vi "MC INIT Mixed Mode.vi"(8 "error in (no error)":errorcluster, 11 "MC VISA resource in":refnum<visa-resource-name>="ASRL1::INSTR") -> (0 "MC error out":errorcluster, 1 "MC Init Complete":bool, 3 "MC VISA resource  out":refnum<visa-resource-name>)   [LabVIEW 2009]
uses:
  <vilib>/Instr/_visa.llb/VISA Configure Serial Port (Instr).vi
panel:
  out "All Stop":bool
  out "Set Mode 3":bool
  in  "Mode command 3":string="^04 C0"
  out "Set Mode 2":bool
  in  "Mode command 2":string="^03 00"
  out "Set RS232 Control":bool
  out "Set Mode 1":bool
  in  "Mode command 1":string="^01 C5"
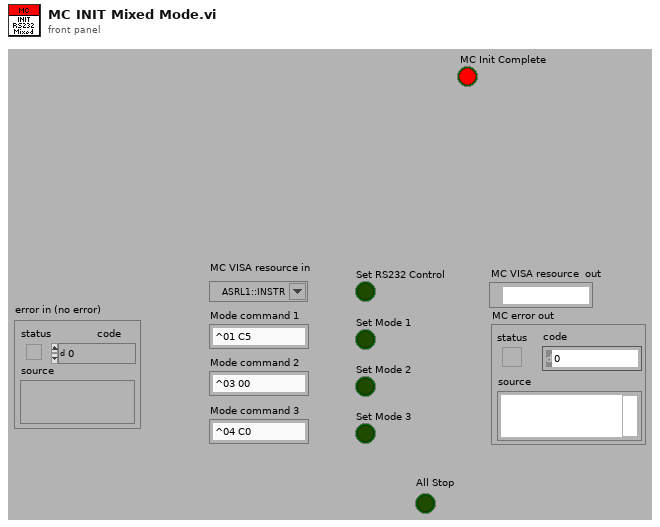
[diagram p1: front panel]
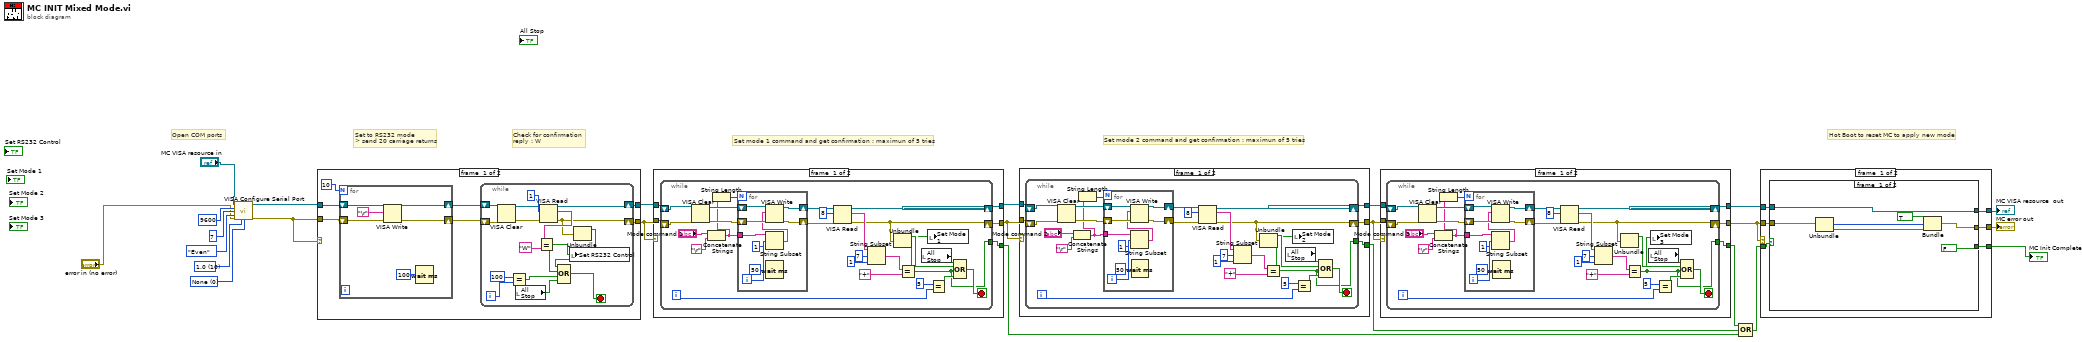
[diagram p0: block diagram]
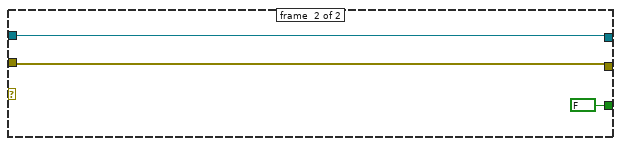
[diagram p2: hidden frame]
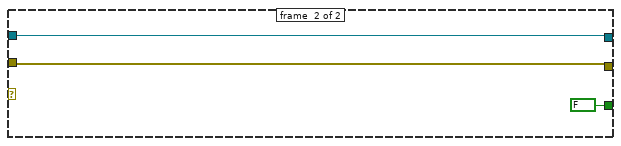
[diagram p3: hidden frame]
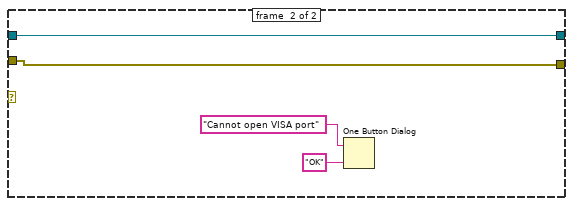
[diagram p4: hidden frame]
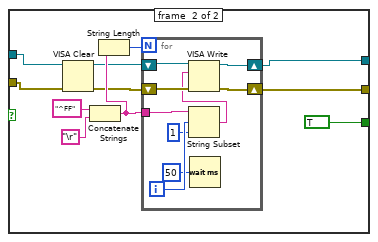
[diagram p5: hidden frame]
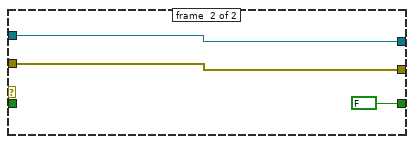
[diagram p6: hidden frame]
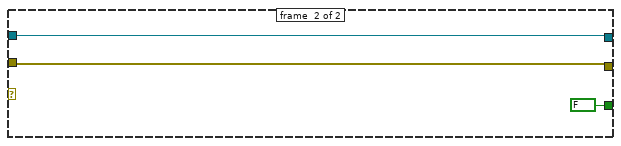
[diagram p7: hidden frame]
diagram:
  w20 = u16 0 items=["None", "XON/XOFF", "RTS/CTS", "XON/XOFF & RTS/CTS", "DTR/DSR", "XON/XOFF & DTR/DSR"] ("flow control (0:none)")
  w21 = u16 10 items=["1.0"=10, "1.5"=15, "2.0"=20] ("stop bits (10: 1 bit)")
  # "Set mode 2 command and get confirmation : maximun of 5 tries"
  # "Hot Boot to reset MC to apply new mode"
  # "Check for confirmation\nreply : W"
  # "Set mode 1 command and get confirmation : maximun of 5 tries"
  # "Set to RS232 mode\n> send 20 carriage returns"
  # "Open COM ports"
  n1 = call-poly "VISA Configure Serial Port"("VISA resource name"="MC VISA resource in", "baud rate (9600)"=u32 9600, "data bits (8)"=u16 7, "parity (0:none)"=enum16{"None", "Odd", "Even", "Mark", "Space"}."Even", "error in (no error)"="error in (no error)", "stop bits (10: 1 bit)"=w21, "flow control (0:none)"=w20) -> ("VISA resource name out"=w19:refnum<visa-resource-name>, "error out"=w15:errorcluster)  [unwired: 7 out]
  n2 = case shown="No Error" w15 {
    tunnel: w15 -> [w30 w56]
    tunnel: w19 -> [w29 w57]
    tunnel: [w28 w57] -> w18
    tunnel: [w25 w56] -> w16
    frame #0 {
      n3 = for {
        N: 10 -> [_]
        shift-right: [w50] -> w27
        shift-left: w30 -> [w53]
        shift-right: [w52] -> w26
        shift-left: w29 -> [w51]
        n4 = VISA Write(VISA resource name=w51, write buffer="\r", error in (no error)=w53) -> (VISA resource name out=w52:refnum<visa-resource-name>, error out=w50:errorcluster)  [unwired: 1 out]
        n5 = Wait (ms)(milliseconds to wait=u32 100) -> ()  [unwired: 1 out]
      }
      n6 = while {
        shift-right: [w43] -> w28
        shift-left: w26 -> [w44]
        shift-right: [w35] -> w25
        shift-left: w27 -> [w42]
        i -> [w39]
        stop <- w36 stop-if-true
        n7 = VISA Clear(VISA resource name=w44, error in (no error)=w42) -> (VISA resource name out=w41:refnum<visa-resource-name>, error out=w34:errorcluster)
        n8 = Equal?(x=100, y=w39) -> (x = y?=w37:bool)
        n9 = local read "All Stop"() -> (w32:bool)
        n10 = VISA Read(VISA resource name=w41, byte count=u32 1, error in (no error)=w34) -> (VISA resource name out=w43:refnum<visa-resource-name>, read buffer=w46:string, error out=w35:errorcluster)  [unwired: 1 out]
        n11 = Equal?(x=w46, y="W") -> (x = y?=w33:bool)
        n12 = local write "Set RS232 Control"(w33) -> ()
        n13 = Unbundle(w35) -> ("status"=w40:bool)  [unwired: 2 out]
        n14 = Compound Arithmetic op=OR(w40, w33, w37, w32) -> (w36:bool)
      }
    }
    frame #1 {
      n15 = One Button Dialog(message="Cannot open VISA port", button name ("OK")="OK") -> ()  [unwired: 1 out]
    }
  }
  n16 = case shown="No Error" w16 {
    tunnel: [w62 w99] -> w11
    tunnel: [w61 w98] -> w12
    tunnel: w18 -> [w60 w99]
    tunnel: w16 -> [w59 w98]
    tunnel: [w58 FALSE] -> w13
    frame #0 {
      n17 = while {
        shift-right: [w83] -> w62
        shift-left: w60 -> [w87]
        shift-right: [w70] -> w61
        shift-left: w59 -> [w86]
        tunnel: [w64] -> w58
        i -> [w67]
        stop <- w65 stop-if-true
        n18 = VISA Clear(VISA resource name=w87, error in (no error)=w86) -> (VISA resource name out=w80:refnum<visa-resource-name>, error out=w79:errorcluster)
        n19 = Concatenate Strings("Mode command 1", "\r") -> (w71:string)
        n20 = String Length(string=w71) -> (length=w72:i32)
        n21 = for {
          N: w72 -> [_]
          tunnel: w71 -> [w92]
          shift-right: [w96] -> w85
          shift-left: w79 -> [w93]
          shift-right: [w95] -> w84
          shift-left: w80 -> [w94]
          i -> [w91]
          n22 = String Subset(string=w92, offset (0)=w91, length (rest)=1 ("length (rest)")) -> (substring=w89:string)
          n23 = VISA Write(VISA resource name=w94, write buffer=w89, error in (no error)=w93) -> (VISA resource name out=w95:refnum<visa-resource-name>, error out=w96:errorcluster)  [unwired: 1 out]
          n24 = Wait (ms)(milliseconds to wait=u32 50) -> ()  [unwired: 1 out]
        }
        n25 = VISA Read(VISA resource name=w84, byte count=u32 8, error in (no error)=w85) -> (VISA resource name out=w83:refnum<visa-resource-name>, read buffer=w76:string, error out=w70:errorcluster)  [unwired: 1 out]
        n26 = String Subset(string=w76, offset (0)=7, length (rest)=1 ("length (rest)")) -> (substring=w75:string)
        n27 = Unbundle(w70) -> ("status"=w66:bool)  [unwired: 2 out]
        n28 = Equal?(x=w75, y="+") -> (x = y?=w64:bool)
        n29 = local read "All Stop"() -> (w63:bool)
        n30 = local write "Set Mode 1"(w64) -> ()
        n31 = Equal?(x=5, y=w67) -> (x = y?=w68:bool)
        n32 = Compound Arithmetic op=OR(w63, w66, w64, w68) -> (w65:bool)
      }
    }
    frame #1 {
    }
  }
  n33 = case shown="No Error" w12 {
    tunnel: [w104 w141] -> w9
    tunnel: [w103 w140] -> w8
    tunnel: w11 -> [w102 w141]
    tunnel: w12 -> [w101 w140]
    tunnel: [w100 FALSE] -> w10
    frame #0 {
      n34 = while {
        shift-right: [w125] -> w104
        shift-left: w102 -> [w129]
        shift-right: [w112] -> w103
        shift-left: w101 -> [w128]
        tunnel: [w106] -> w100
        i -> [w109]
        stop <- w107 stop-if-true
        n35 = VISA Clear(VISA resource name=w129, error in (no error)=w128) -> (VISA resource name out=w122:refnum<visa-resource-name>, error out=w121:errorcluster)
        n36 = Concatenate Strings("Mode command 2", "\r") -> (w113:string)
        n37 = String Length(string=w113) -> (length=w114:i32)
        n38 = for {
          N: w114 -> [_]
          tunnel: w113 -> [w134]
          shift-right: [w138] -> w127
          shift-left: w121 -> [w135]
          shift-right: [w137] -> w126
          shift-left: w122 -> [w136]
          i -> [w133]
          n39 = String Subset(string=w134, offset (0)=w133, length (rest)=1 ("length (rest)")) -> (substring=w131:string)
          n40 = VISA Write(VISA resource name=w136, write buffer=w131, error in (no error)=w135) -> (VISA resource name out=w137:refnum<visa-resource-name>, error out=w138:errorcluster)  [unwired: 1 out]
          n41 = Wait (ms)(milliseconds to wait=u32 50) -> ()  [unwired: 1 out]
        }
        n42 = VISA Read(VISA resource name=w126, byte count=u32 8, error in (no error)=w127) -> (VISA resource name out=w125:refnum<visa-resource-name>, read buffer=w118:string, error out=w112:errorcluster)  [unwired: 1 out]
        n43 = String Subset(string=w118, offset (0)=7, length (rest)=1 ("length (rest)")) -> (substring=w117:string)
        n44 = Unbundle(w112) -> ("status"=w108:bool)  [unwired: 2 out]
        n45 = Equal?(x=w117, y="+") -> (x = y?=w106:bool)
        n46 = local read "All Stop"() -> (w105:bool)
        n47 = local write "Set Mode 2"(w106) -> ()
        n48 = Equal?(x=5, y=w109) -> (x = y?=w110:bool)
        n49 = Compound Arithmetic op=OR(w105, w108, w106, w110) -> (w107:bool)
      }
    }
    frame #1 {
    }
  }
  n50 = case shown="No Error" w8 {
    tunnel: [w146 w183] -> w7
    tunnel: [w145 w182] -> w5
    tunnel: w9 -> [w144 w183]
    tunnel: w8 -> [w143 w182]
    tunnel: [w142 FALSE] -> w6
    frame #0 {
      n51 = while {
        shift-right: [w167] -> w146
        shift-left: w144 -> [w171]
        shift-right: [w154] -> w145
        shift-left: w143 -> [w170]
        tunnel: [w148] -> w142
        i -> [w151]
        stop <- w149 stop-if-true
        n52 = VISA Clear(VISA resource name=w171, error in (no error)=w170) -> (VISA resource name out=w164:refnum<visa-resource-name>, error out=w163:errorcluster)
        n53 = Concatenate Strings("Mode command 3", "\r") -> (w155:string)
        n54 = String Length(string=w155) -> (length=w156:i32)
        n55 = for {
          N: w156 -> [_]
          tunnel: w155 -> [w176]
          shift-right: [w180] -> w169
          shift-left: w163 -> [w177]
          shift-right: [w179] -> w168
          shift-left: w164 -> [w178]
          i -> [w175]
          n56 = String Subset(string=w176, offset (0)=w175, length (rest)=1 ("length (rest)")) -> (substring=w173:string)
          n57 = VISA Write(VISA resource name=w178, write buffer=w173, error in (no error)=w177) -> (VISA resource name out=w179:refnum<visa-resource-name>, error out=w180:errorcluster)  [unwired: 1 out]
          n58 = Wait (ms)(milliseconds to wait=u32 50) -> ()  [unwired: 1 out]
        }
        n59 = VISA Read(VISA resource name=w168, byte count=u32 8, error in (no error)=w169) -> (VISA resource name out=w167:refnum<visa-resource-name>, read buffer=w160:string, error out=w154:errorcluster)  [unwired: 1 out]
        n60 = String Subset(string=w160, offset (0)=7, length (rest)=1 ("length (rest)")) -> (substring=w159:string)
        n61 = Unbundle(w154) -> ("status"=w150:bool)  [unwired: 2 out]
        n62 = Equal?(x=w159, y="+") -> (x = y?=w148:bool)
        n63 = local read "All Stop"() -> (w147:bool)
        n64 = local write "Set Mode 3"(w148) -> ()
        n65 = Equal?(x=5, y=w151) -> (x = y?=w152:bool)
        n66 = Compound Arithmetic op=OR(w147, w150, w148, w152) -> (w149:bool)
      }
    }
    frame #1 {
    }
  }
  n67 = Compound Arithmetic op=OR(w6, w10, w13) -> (w14:bool)
  n68 = case shown="No Error" w5 {
    tunnel: w5 -> [w189 w219]
    tunnel: w7 -> [w188 w218]
    tunnel: w14 -> [w185 _]
    tunnel: [w187 w219] -> w3
    tunnel: [w186 w218] -> w4
    tunnel: [w184 FALSE] -> w2
    frame #0 {
      n69 = case shown="False" w185 {
        tunnel: w189 -> [w195 w201]
        tunnel: w188 -> [w191 w200]
        tunnel: [w196 w199] -> w187
        tunnel: [w191 w198] -> w186
        tunnel: [FALSE TRUE] -> w184
        frame #0 {
          n70 = Unbundle(w195) -> ("code"=w193:i32, "source"=w194:string)  [unwired: 1 out]
          n71 = Bundle(TRUE, "code"=w193, "source"=w194) -> (w196:cluster{bool, "code":i32, "source":string})  [unwired: 1 out]
        }
        frame #1 {
          n72 = VISA Clear(VISA resource name=w200, error in (no error)=w201) -> (VISA resource name out=w204:refnum<visa-resource-name>, error out=w205:errorcluster)
          n73 = Concatenate Strings("^FF" ("string"), "\r") -> (w207:string)
          n74 = String Length(string=w207) -> (length=w206:i32)
          n75 = for {
            N: w206 -> [_]
            tunnel: w207 -> [w212]
            shift-right: [w216] -> w199
            shift-left: w205 -> [w213]
            shift-right: [w215] -> w198
            shift-left: w204 -> [w214]
            i -> [w211]
            n76 = String Subset(string=w212, offset (0)=w211, length (rest)=1 ("length (rest)")) -> (substring=w209:string)
            n77 = VISA Write(VISA resource name=w214, write buffer=w209, error in (no error)=w213) -> (VISA resource name out=w215:refnum<visa-resource-name>, error out=w216:errorcluster)  [unwired: 1 out]
            n78 = Wait (ms)(milliseconds to wait=u32 50) -> ()  [unwired: 1 out]
          }
        }
      }
    }
    frame #1 {
    }
  }
  "MC VISA resource  out" <- w4
  "MC error out" <- w3
  "MC Init Complete" <- w2
